vi "New Entry.vi"(6 "Time Stamp (Now)":timestamp, 10 "New Entry":string[](array[string]) caption="New Entry (Table Row)", 11 "Cyclic Table in":refnum<class "Cyclic Table.lvclass">) -> (3 "Cyclic Table out":refnum<class "Cyclic Table.lvclass">)   [LabVIEW 2024, in "Cyclic Table.lvclass"]
doc: "Add a new row entry to the cyclic table, overwriting (if necessary) the oldest previous entry."
uses:
  Cyclic Table.lvclass
  Cyclic Table.lvclass/Cyclic Table.ctl
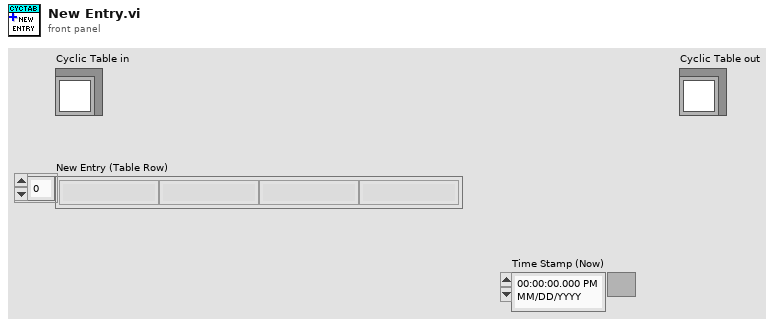
[diagram p1: front panel]
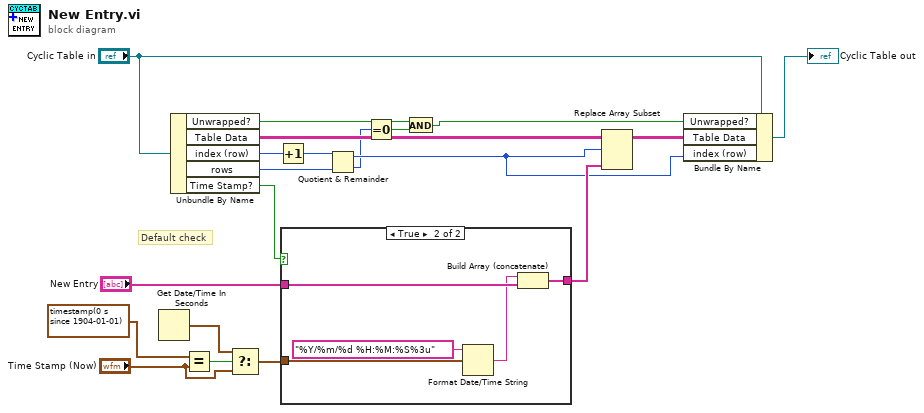
[diagram p0: block diagram]
diagram:
  # "Default check"
  n1 = Get Date/Time In Seconds() -> (seconds since 1Jan1904=w16:timestamp)
  n2 = Unbundle By Name("Cyclic Table in") -> ("Unwrapped?"=w3:bool, "Table Data"=w7:string[][], "index (row)"=w18:i32, "rows"=w6:i32, "Time Stamp?"=w11:bool)
  n3 = Equal?(x=timestamp(0 s since 1904-01-01) ("y"), y="Time Stamp (Now)") -> (x = y?=w15:bool)
  n4 = Select(t=w16, s=w15, f="Time Stamp (Now)") -> (s? t:f=w14:timestamp)
  n5 = Increment(x=w18) -> (x+1=w8:i32)
  n6 = case shown="True" w11 {
    tunnel: w14 -> [_ w23]
    tunnel: "New Entry" -> [w21 w26]
    tunnel: [w21 w25] -> w9
    frame False {
    }
    frame True {
      n7 = Format Date/Time String(time format string (%c)="%Y/%m/%d %H:%M:%S%3u", seconds (now)=w23) -> (date/time string=w22:string)  [unwired: 1 in]
      n8 = Build Array (concatenate)(w22, w26) -> (w25:string[])
    }
  }
  n9 = Quotient & Remainder(x=w8, y=w6) -> (x-y*floor(x/y)=w5:i32, floor(x/y)=w2:i32)
  n10 = Equal To 0?(x=w2) -> (x = 0?=w1:bool)
  n11 = And(x=w3, y=w1) -> (x .and. y?=w4:bool)
  n12 = Replace Array Subset(array=w7, new element=w9, index (row)=w5) -> (w17:string[][])  [unwired: 1 in]
  n13 = Bundle By Name(cluster="Cyclic Table in", "Unwrapped?"=w4, "Table Data"=w17, "index (row)"=w5) -> (→"Cyclic Table out":refnum<class "Cyclic Table.lvclass">)
